vi "CheckDuplicateData.vi"(8 "error in (no error)":errorcluster, 10 "ToCheck in":refnum<data-value>, 11 "LLNode in":refnum<class "LLNode.lvclass">) -> (0 "error out":errorcluster, 1 "IsDuplicate":bool, 2 "ToCheck out":refnum<data-value>, 3 "LLNode out":refnum<class "LLNode.lvclass">)   [LabVIEW 2014, in "LinkedList.lvlib" / "LLNode.lvclass"]
doc: "Dynamic Dispatch placeholder used in to determine if two nodes in the linked list have the same data. Used in the DataIsInList method."
uses:
  <userlib>/AdvancedDataStructures/ClassBased/LLNode/LLNode.lvclass
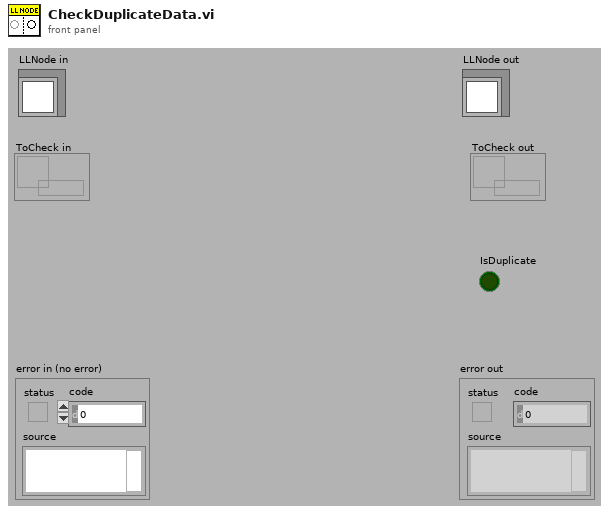
[diagram p1: front panel]
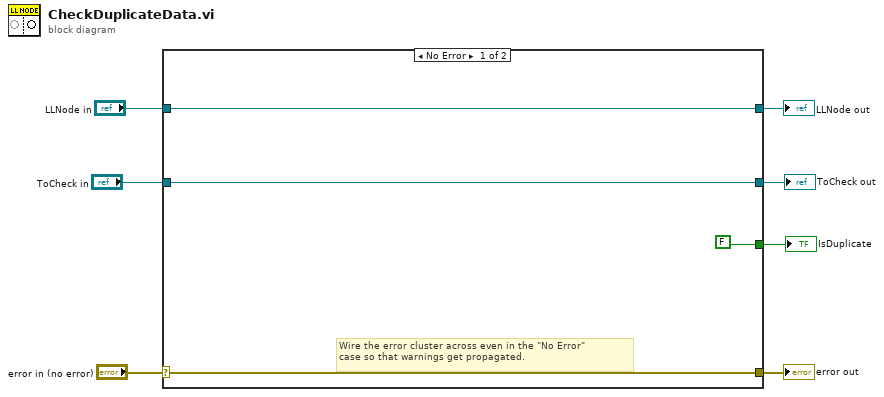
[diagram p0: block diagram]
diagram:
  n1 = case shown="No Error" "error in (no error)" {
    selector: "error in (no error)" -> [w10 w14]
    tunnel: [w10 w14] -> w6
    tunnel: [w11 w13] -> w4
    tunnel: "LLNode in" -> [w11 w13]
    tunnel: "ToCheck in" -> [w9 w12]
    tunnel: [w9 w12] -> w2
    tunnel: [FALSE ("IsDuplicate") _] -> w1
    frame No Error {
      # "Wire the error cluster across even in the \"No Error\"\ncase so that warnings get propagated."
    }
    frame Error {
    }
  }
  "error out" <- w6
  "LLNode out" <- w4
  "ToCheck out" <- w2
  "IsDuplicate" <- w1
